vi "HIOKI PW3390 WAI.vi"(8 "error in (no error)":errorcluster, 11 "VISA Resource":refnum<visa-resource-name>) -> (0 "error out":errorcluster, 3 "VISA Resource out":refnum<visa-resource-name>)   [LabVIEW 2009]
doc: "Waits until the next refresh is completed.\n\n<B>Note</B>\nIn Hold status, the display data will not change even when this command is executed."
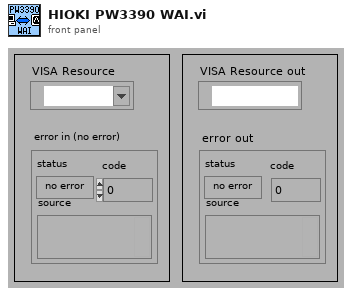
[diagram p1: front panel]
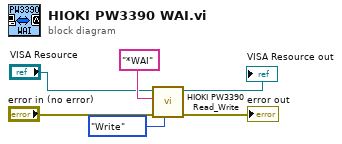
[diagram p0: block diagram]
diagram:
  n1 = call <instrlib>:"HIOKI PW3390 Read_Write.vi"("Read/Write"=enum16{"Read", "Write"}."Write", "error in (no error)"="error in (no error)", "data in"="*WAI", "VISA Resource"="VISA Resource") -> ("error out"=→"error out":errorcluster, "VISA Resource out"=→"VISA Resource out":refnum<visa-resource-name>)  [unwired: 5 in, 1 out]
